vi "CODCr通讯.vi"() -> ()   [LabVIEW 2016, in "CODCr库.lvlib"]
uses:
  <vilib>/NI/Modbus Library/API/Wrapper/Create TCP Slave.vi
  <vilib>/NI/Modbus Library/API/slave/Modbus Slave.lvclass
  <vilib>/Plasmionique/MB Master/MB_Master/MB_Master.lvclass
  <vilib>/Plasmionique/MB Master/MB Master.lvlib
  <vilib>/Utility/config.llb/NI_LVConfig.lvlib
  <vilib>/NI/Modbus Library/API/Wrapper/API Main.lvlib
panel:
  out "状态告警区":u16[](array[numeric])
  out "测量数据区":u16[](array[numeric])
  in  "读取参数":bool
  in  "读取数据":bool
  in  "释放串口":bool
  in  "打开串口":bool
  out "队列中元素数量":i32
  out "元素":cluster{"命令":string}[](array[cluster])
  out "待处理插入数量":i32
  out "读取公式":u16[](array[numeric])
  out "读取参数":u16[](array[numeric])
  out "数据存储":u16[](array[numeric])
  out "通讯状态":bool
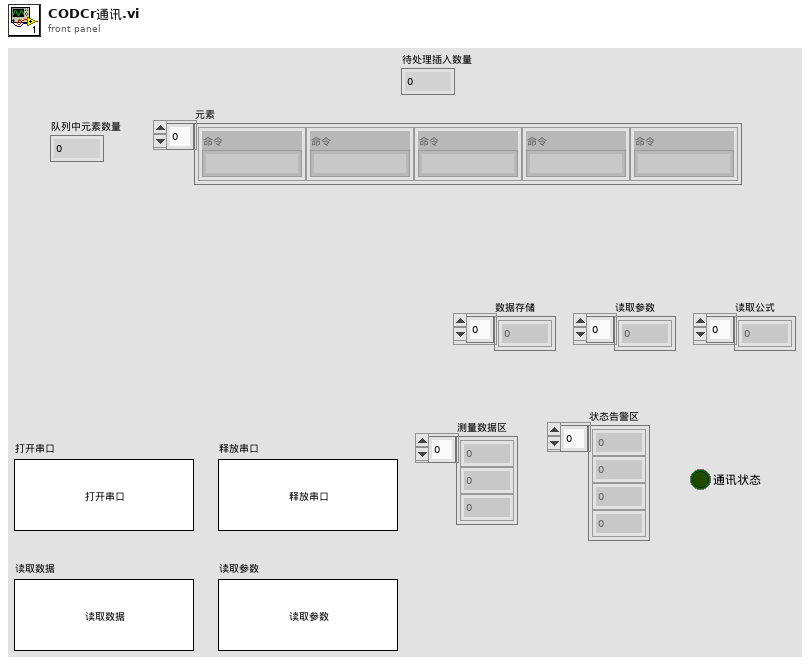
[diagram p1: front panel]
types:
  T1 = typedef "NI_LVConfig.lvlib/Config Data RefNum.ctl" = refnum<k1>
  T2 = cluster{"因子编码":u32, "单位":u16, "标样参考值":sgl, "水样数据时间":timestamp, "水样实测值":sgl, "水样数据标识":string, "标样数据时间":timestamp, "标样实测值":sgl, "标样数据标识":string, "空白数据时间":timestamp, "空白实测值":sgl, "空白数据标识":string, "零点核查数据时间":timestamp, "零点核查实测值":sgl, "零点核查数据标识":string, "跨度核查数据时间":timestamp, "跨度核查实测值":sgl, "跨度核查数据标识":string, "加标回收数据时间":timestamp, "加标回收实测值":sgl, "加标回收数据标识":string, "平行样数据时间":timestamp, "平行样实测值":sgl, "平行样数据标识":string}
  T3 = cluster{"系统时间":timestamp, "工作状态":enum16{"空闲", "水样测试", "标样核查", "零点核查", "跨度核查", "空白测试", "平行样测试", "加标回收", "空白校准", "标样校准", "初始化（清洗）"}, "测量模式":enum16{"待机", "连续模式", "周期模式", "定点模式", "受控模式", "手动模式"}, "告警代码":u16, "故障代码":u16, "日志代码":u16, "软件版本":u16, "F0":sgl, "F1":sgl, "F2":sgl, "F3":sgl, "T":sgl, "H":sgl, "id":u16, "flowid":u16, "量程":u16}
  T4 = cluster{"测量精度":u16, "消解温度":u16, "消解时长":u16, "量程下限":sgl, "量程上限":sgl, "曲线斜率K":sgl, "曲线斜率B":sgl, "标定日期":timestamp, "标液1浓度":sgl, "标液1测量过程值":sgl, "标液2浓度":sgl, "标液2测量过程值":sgl, "标液3浓度":sgl, "标液3测量过程值":sgl, "标液4浓度":sgl, "标液4测量过程值":sgl, "标液5浓度":sgl, "标液5测量过程值":sgl, "线性相关系数":sgl, "试剂余量":u32, "测量滴定值或吸光度":sgl, "空白校准时间":timestamp, "标样校准时间":timestamp, "检出限值":sgl, "校准系数":sgl, "设备系列号":string}
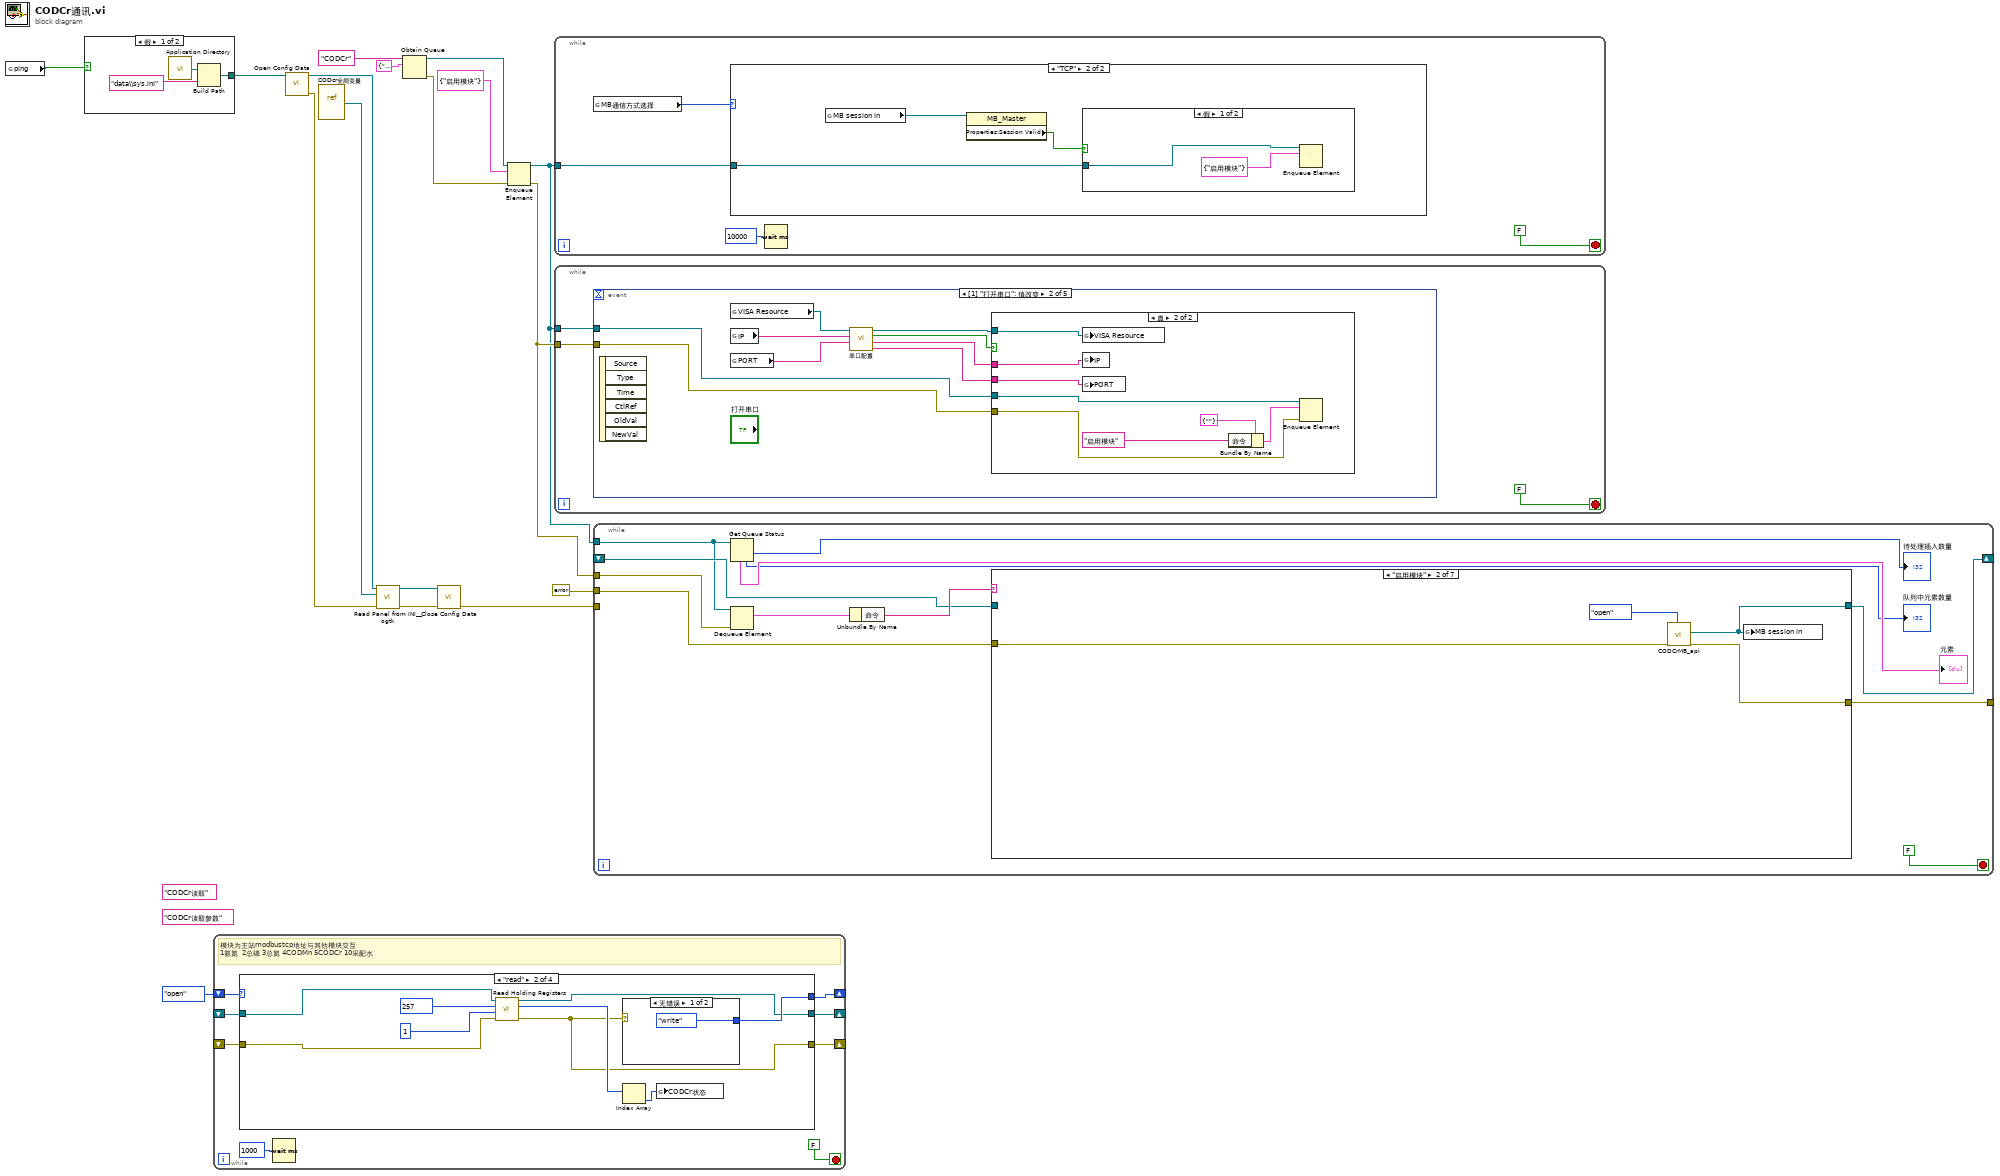
[diagram p0: block diagram]
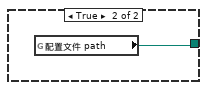
[diagram p2: hidden frame]
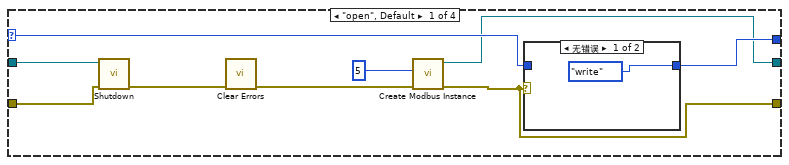
[diagram p5: hidden frame]
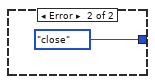
[diagram p7: hidden frame]
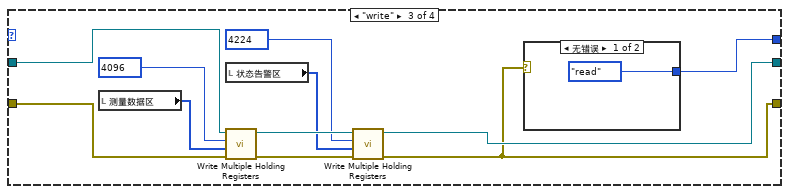
[diagram p8: hidden frame]
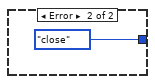
[diagram p9: hidden frame]
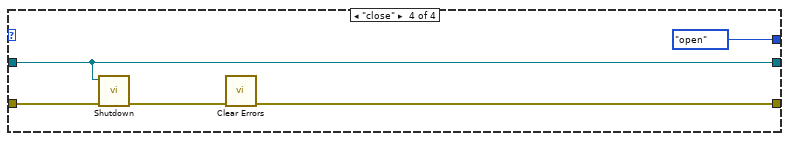
[diagram p10: hidden frame]
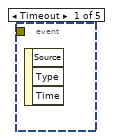
[diagram p11: hidden frame]
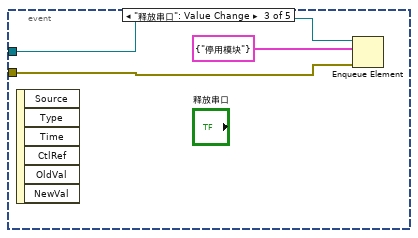
[diagram p13: hidden frame]
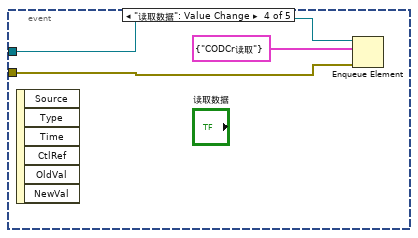
[diagram p14: hidden frame]
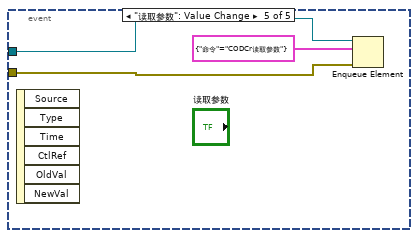
[diagram p15: hidden frame]
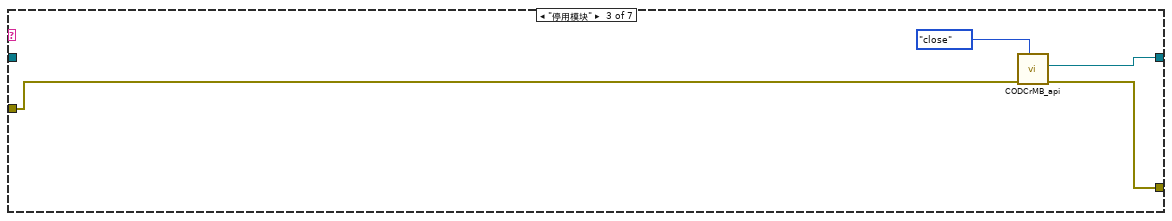
[diagram p17: hidden frame]
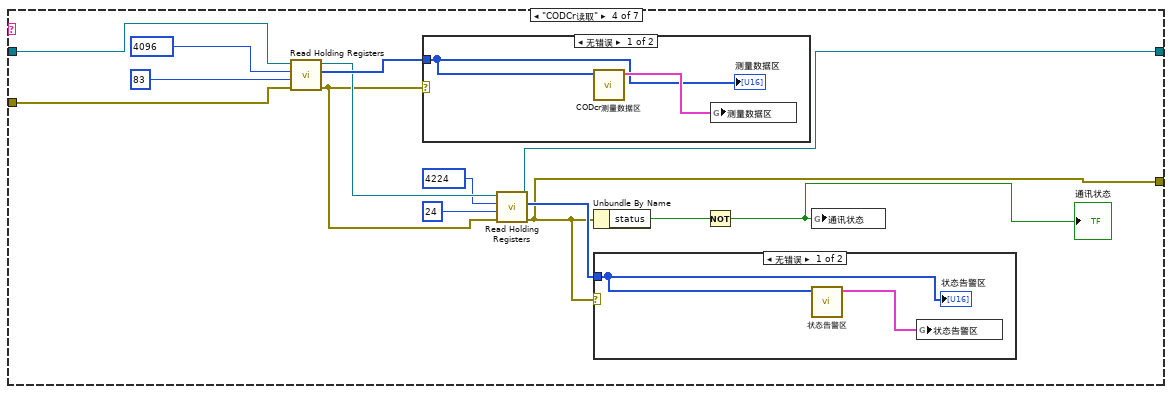
[diagram p18: hidden frame]
diagram:
  (unwired) "CODCr读取参数" ("名称（未命名）")
  (unwired) "CODCr读取" ("名称（未命名）")
  n1 = global read "CODcr全局变量.vi" "ping"() -> (w2:bool)
  n2 = case shown="假" w2 {
    tunnel: [w19 w21] -> w1
    frame False {
      n3 = call <vilib>:"Application Directory.vi"() -> ("Application Directory"=w20:path)
      n4 = Build Path(base path=w20, name or relative path="data\\sys.ini" ("名称或相对路径")) -> (appended path=w19:path)
    }
    frame True {
      n5 = global read "CODcr全局变量.vi" "配置文件 path"() -> (w21:path)
    }
  }
  n6 = while {
    shift-right: [w27] -> _
    shift-left: _ -> [w29]
    shift-right: [w26] -> _
    shift-left: _ -> [w28]
    shift-right: [w23] -> _
    shift-left: enum16{"open", "read", "write", "close"}."open" -> [w24]
    stop <- FALSE stop-if-true
    # "模块为主站modbustcp地址与其他模块交互\n1氨氮  2总磷 3总氮 4CODMn 5CODCr 10采配水"
    n7 = case shown="\"read\"" w24 {
      selector: w24 -> [w38 _ _ _]
      tunnel: w29 -> [w32 w44 w61 w67]
      tunnel: w28 -> [w31 w43 w57 w66]
      tunnel: [w35 w41 w53 w67] -> w27
      tunnel: [w34 w42 w52 w69] -> w26
      tunnel: [w37 w49 w62 enum16{"open", "read", "write", "close"}."open"] -> w23
      frame "open", Default {
        n8 = call-dynamic "Shutdown.vi"("error in"=w31, "Modbus slave in"=w32) -> ("error out"=w30:errorcluster)  [unwired: 9 in]
        n9 = call <vilib>:"Clear Errors.vi"("error in (no error)"=w30) -> ("error out"=w33:errorcluster)  [unwired: 5 in, 1 out]
        n10 = call-poly <vilib>:"Create Modbus Instance.vi"("error in"=w33, "port (502)"=u16 5) -> ("error out"=w34:errorcluster, "TCP slave instance"=w35:refnum<class "Modbus Slave.lvclass">)  [unwired: 8 in]
        n11 = case shown="无错误" w34 {
          tunnel: w38 -> [_ w40]
          tunnel: [enum16{"open", "read", "write", "close"}."write" w40] -> w37
          frame No Error {
          }
          frame Error {
          }
        }
      }
      frame "read" {
        n12 = call-dynamic <vilib>:"Read Holding Registers.vi"("error in"=w43, "number of inputs"=u16 1, "starting address"=u16 257, "Modbus slave in"=w44) -> ("error out"=w42:errorcluster, "register values"=w46:u16[], "Modbus slave out"=w41:refnum<class "Modbus Slave.lvclass">)  [unwired: 5 in]
        n13 = case shown="无错误" w42 {
          tunnel: [enum16{"open", "read", "write", "close"}."write" enum16{"open", "read", "write", "close"}."close"] -> w49
          frame No Error {
          }
          frame Error {
          }
        }
        n14 = Index Array(array=w46) -> (element=w45:u16)  [unwired: 1 in]
        n15 = global write "CODCr外部API.vi" "CODCr状态"(w45) -> ()
      }
      frame "write" {
        n16 = local read "测量数据区"() -> (w59:u16[])
        n17 = local read "状态告警区"() -> (w54:u16[])
        n18 = call-dynamic "Write Multiple Holding Registers.vi"("error in"=w57, "registers to write"=w59, "starting address"=u16 4096, "Modbus slave in"=w61) -> ("error out"=w56:errorcluster, "Modbus slave out"=w58:refnum<class "Modbus Slave.lvclass">)  [unwired: 6 in]
        n19 = call-dynamic "Write Multiple Holding Registers.vi"("error in"=w56, "registers to write"=w54, "starting address"=u16 4224, "Modbus slave in"=w58) -> ("error out"=w52:errorcluster, "Modbus slave out"=w53:refnum<class "Modbus Slave.lvclass">)  [unwired: 6 in]
        n20 = case shown="无错误" w52 {
          tunnel: [enum16{"open", "read", "write", "close"}."read" enum16{"open", "read", "write", "close"}."close"] -> w62
          frame No Error {
          }
          frame Error {
          }
        }
      }
      frame "close" {
        n21 = call-dynamic "Shutdown.vi"("error in"=w66, "Modbus slave in"=w67) -> ("error out"=w65:errorcluster)  [unwired: 9 in]
        n22 = call <vilib>:"Clear Errors.vi"("error in (no error)"=w65) -> ("error out"=w69:errorcluster)  [unwired: 5 in, 1 out]
      }
    }
    n23 = Wait (ms)(milliseconds to wait=u32 1000 ("等待时间（毫秒）")) -> ()  [unwired: 1 out]
  }
  n24 = call <vilib>:"Open Config Data.vi"("configuration file path"=w1) -> ("error out"=w8:errorcluster, "refnum"=w11:T1)  [unwired: 8 in, 1 out]
  n25 = vi-ref "CODcr全局变量.vi"() -> (w10:refnum<vi>)
  n26 = call <userlib>:"Read Panel from INI__ogtk.vi"("error in (no error)"=w8, "VI ref"=w10, "refnum"=w11) -> ("error out"=w7:errorcluster, "refnum out"=w9:T1)  [unwired: 7 in]
  n27 = Obtain Queue(name (unnamed)="CODCr" ("名称（未命名）"), element data type=cluster{"命令":string} {"命令"="启用模块"} ("元素")) -> (queue out=w14:refnum<queue>, error out=w13:errorcluster)  [unwired: 3 in, 1 out]
  n28 = call <vilib>:"Close Config Data.vi"("error in (no error)"=w7, "refnum"=w9) -> ("error out"=w3:errorcluster)  [unwired: 8 in, 1 out]
  n29 = Enqueue Element(queue=w14, element=cluster{"命令":string} {"命令"="启用模块"} ("元素"), error in (no error)=w13) -> (queue out=w4:refnum<queue>, error out=w6:errorcluster)  [unwired: 1 in, 1 out]
  n30 = while {
    tunnel: w4 -> [w73]
    stop <- FALSE stop-if-true
    n31 = global read "CODcr全局变量.vi" "MB通信方式选择"() -> (w71:enum16{"串口", "TCP"})
    n32 = case shown="\"TCP\"" w71 {
      tunnel: w73 -> [_ w74]
      frame "串口", Default {
      }
      frame "TCP" {
        n33 = global read "CODCr外部API.vi" "MB session in"() -> (w76:refnum<class "MB_Master.lvclass">)
        n34 = property class="MB_Master"(reference=w76) -> ("Properties:Session Valid"=w75:bool)  [unwired: 1 in, 2 out]
        n35 = case shown="假" w75 {
          tunnel: w74 -> [w78 _]
          frame False {
            n36 = Enqueue Element(queue=w78, element=cluster{"命令":string} {"命令"="启用模块"} ("元素")) -> ()  [unwired: 2 in, 3 out]
          }
          frame True {
          }
        }
      }
    }
    n37 = Wait (ms)(milliseconds to wait=u32 10000 ("等待时间（毫秒）")) -> ()  [unwired: 1 out]
  }
  n38 = while {
    tunnel: w4 -> [w80]
    tunnel: w6 -> [w79]
    stop <- FALSE stop-if-true
    n39 = event shown="[1] \"打开串口\": 值改变" {
      selector: _ -> [_ _ _ _ _]
      dyn-events: _ -> [_ _ _ _ _]
      timeout: _ -> [_ _ _ _ _]
      tunnel: w80 -> [_ w90 w101 w103 w106]
      tunnel: w79 -> [_ w89 w100 w102 w105]
      event Timeout {
        n40 = event-data() -> ()  [unwired: 1 in, 3 out]
      }
      event "打开串口": Value Change {
        n41 = event-data() -> ()  [unwired: 1 in, 6 out]
        n42 = global read "CODcr全局变量.vi" "VISA Resource"() -> (w88:refnum<visa-resource-name>)
        n43 = global read "CODcr全局变量.vi" "IP"() -> (w83:string)
        n44 = global read "CODcr全局变量.vi" "PORT"() -> (w82:string)
        n45 = call "串口配置.vi"("PORT"=w82, "IP"=w83, "请选择串口:"=w88) -> ("PORT 2"=w84:string, "IP 2"=w85:string, "确认 2"=w87:bool, "VISA资源名称 2"=w86:refnum<visa-resource-name>)  [unwired: 5 in]
        n46 = case shown="真" w87 {
          tunnel: w86 -> [_ w93]
          tunnel: w90 -> [_ w95]
          tunnel: w89 -> [_ w94]
          tunnel: w85 -> [_ w92]
          tunnel: w84 -> [_ w91]
          frame False {
          }
          frame True {
            n47 = global write "CODcr全局变量.vi" "VISA Resource"(w93) -> ()
            n48 = global write "CODcr全局变量.vi" "IP"(w92) -> ()
            n49 = global write "CODcr全局变量.vi" "PORT"(w91) -> ()
            n50 = Bundle By Name(cluster=cluster{"命令":string} {"命令"=""} ("元素"), "命令"="启用模块" ("名称（未命名）")) -> (w96:cluster{"命令":string})
            n51 = Enqueue Element(queue=w95, element=w96, error in (no error)=w94) -> ()  [unwired: 1 in, 3 out]
          }
        }
      }
      event "释放串口": Value Change {
        n52 = event-data() -> ()  [unwired: 1 in, 6 out]
        n53 = Enqueue Element(queue=w101, element=cluster{"命令":string} {"命令"="停用模块"} ("元素"), error in (no error)=w100) -> ()  [unwired: 1 in, 3 out]
      }
      event "读取数据": Value Change {
        n54 = event-data() -> ()  [unwired: 1 in, 6 out]
        n55 = Enqueue Element(queue=w103, element=cluster{"命令":string} {"命令"="CODCr读取"} ("元素"), error in (no error)=w102) -> ()  [unwired: 1 in, 3 out]
      }
      event "读取参数": Value Change {
        n56 = event-data() -> ()  [unwired: 1 in, 6 out]
        n57 = Enqueue Element(queue=w106, element=cluster{"命令":string} {"命令"="CODCr读取参数"} ("元素"), error in (no error)=w105) -> ()  [unwired: 1 in, 3 out]
      }
    }
  }
  n58 = while {
    tunnel: w4 -> [w111]
    tunnel: w6 -> [w118]
    tunnel: [w112] -> _
    shift-right: [w115] -> _
    shift-left: _ -> [w114]
    tunnel: errorcluster {"status"=FALSE, "code"=0, "source"=""} ("error out") -> [w113]
    tunnel: w3 -> [_]
    stop <- FALSE stop-if-true
    n59 = Get Queue Status(queue=w111) -> (# pending insert=→"待处理插入数量":i32, # elements in queue=→"队列中元素数量":i32, elements=→"元素":cluster{"命令":string}[])  [unwired: 2 in, 5 out]
    n60 = Dequeue Element(queue=w111, error in (no error)=w118) -> (element=w117:cluster{"命令":string})  [unwired: 1 in, 3 out]
    n61 = Unbundle By Name(w117) -> ("命令"=w116:string)
    n62 = case shown="\"启用模块\"" w116 {
      tunnel: [w121 w122 w126 w137 w150 w158 w167] -> w115
      tunnel: [w120 w125 w127 w130 w148 w157 w166] -> w112
      tunnel: w114 -> [w121 _ _ w143 w154 w161 w170]
      tunnel: w113 -> [w120 w123 w128 w142 w151 w160 w169]
      frame Default {
      }
      frame "启用模块" {
        n63 = call "CODCrMB_api.vi"("STEP"=enum16{"open", "read", "write", "close"}."open", "Error in"=w123) -> ("error out"=w125:errorcluster, "MB session out"=w122:refnum<class "MB_Master.lvclass">)  [unwired: 7 in, 1 out]
        n64 = global write "CODCr外部API.vi" "MB session in"(w122) -> ()
      }
      frame "停用模块" {
        n65 = call "CODCrMB_api.vi"("STEP"=enum16{"open", "read", "write", "close"}."close", "Error in"=w128) -> ("error out"=w127:errorcluster, "MB session out"=w126:refnum<class "MB_Master.lvclass">)  [unwired: 7 in, 1 out]
      }
      frame "CODCr读取" {
        n66 = call <vilib>:"Read Holding Registers.vi"("error in (no error)"=w142, "quantity"=u16 83 ("number of holding registers"), "starting address"=u16 4096, "MB session in"=w143) -> ("error out"=w139:errorcluster, "Registers"=w141:u16[], "MB session out"=w140:refnum<class "MB_Master.lvclass">)  [unwired: 5 in]
        n67 = case shown="无错误" w139 {
          tunnel: w141 -> [w146 _]
          frame No Error {
            n68 = call "CODcr测量数据区.vi"("数组"=w146) -> ("测量数据区"=w147:T2)  [unwired: 10 in]
            n69 = global write "CODcr全局变量.vi" "测量数据区"(w147) -> ()
            "测量数据区" <- w146
          }
          frame Error {
          }
        }
        n70 = call <vilib>:"Read Holding Registers.vi"("error in (no error)"=w139, "quantity"=u16 24 ("number of holding registers"), "starting address"=u16 4224, "MB session in"=w140) -> ("error out"=w130:errorcluster, "Registers"=w138:u16[], "MB session out"=w137:refnum<class "MB_Master.lvclass">)  [unwired: 5 in]
        n71 = Unbundle By Name(w130) -> ("status"=w131:bool)
        n72 = case shown="无错误" w130 {
          tunnel: w138 -> [w144 _]
          frame No Error {
            n73 = call "状态告警区.vi"("数组"=w144) -> ("状态告警区"=w145:T3)  [unwired: 10 in]
            n74 = global write "CODcr全局变量.vi" "状态告警区"(w145) -> ()
            "状态告警区" <- w144
          }
          frame Error {
          }
        }
        n75 = Not(x=w131) -> (.not. x?=w132:bool)
        "通讯状态" <- w132
        n76 = global write "CODcr全局变量.vi" "通讯状态"(w132) -> ()
      }
      frame "CODMn读取写入DATABASE" {
        n77 = call <vilib>:"Read Holding Registers.vi"("error in (no error)"=w151, "quantity"=u16 10 ("number of holding registers"), "starting address"=u16 4101, "MB session in"=w154) -> ("error out"=w148:errorcluster, "Registers"=w149:u16[], "MB session out"=w150:refnum<class "MB_Master.lvclass">)  [unwired: 5 in]
        n78 = case shown="无错误" w148 {
          tunnel: w149 -> [_ _]
          frame No Error {
          }
          frame Error {
          }
        }
      }
      frame "CODCr读取参数" {
        n79 = call <vilib>:"Read Holding Registers.vi"("error in (no error)"=w160, "quantity"=u16 19 ("number of holding registers"), "starting address"=u16 4256, "MB session in"=w161) -> ("error out"=w157:errorcluster, "Registers"=w159:u16[], "MB session out"=w158:refnum<class "MB_Master.lvclass">)  [unwired: 5 in]
        n80 = case shown="无错误" w157 {
          tunnel: w159 -> [w162 _]
          frame No Error {
            n81 = call "关键参数区.vi"("数组"=w162) -> ("关键参数区"=w163:T4)  [unwired: 10 in]
            n82 = global write "CODcr全局变量.vi" "关键参数区"(w163) -> ()
          }
          frame Error {
          }
        }
      }
      frame "CODMn读取公式" {
        n83 = call <vilib>:"Read Holding Registers.vi"("error in (no error)"=w169, "quantity"=u16 94 ("number of holding registers"), "starting address"=u16 4616, "MB session in"=w170) -> ("error out"=w166:errorcluster, "Registers"=w168:u16[], "MB session out"=w167:refnum<class "MB_Master.lvclass">)  [unwired: 5 in]
        n84 = case shown="无错误" w166 {
          tunnel: w168 -> [_ _]
          frame No Error {
          }
          frame Error {
          }
        }
      }
    }
  }
